vi "Load LV Class from Disk.vi"(8 "error in":errorcluster, 11 "Class Path":path) -> (0 "error out":errorcluster, 3 "Object Out":refnum<class>)   [LabVIEW 2015, in "Configuration Tool.lvlib"]
uses:
  Configuration Tool.lvlib
  <vilib>/NI/Configuration Framework/class discovery singleton/class discovery singleton.lvlib
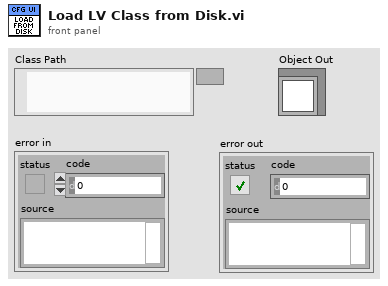
[diagram p1: front panel]
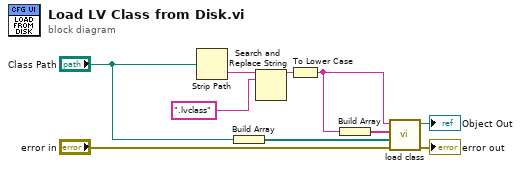
[diagram p0: block diagram]
diagram:
  n1 = Strip Path(path="Class Path") -> (name=w3:string)  [unwired: 1 out]
  n2 = Build Array("Class Path") -> (w5:path[])
  n3 = Search and Replace String(input string=w3, search string=".lvclass") -> (result string=w8:string)  [unwired: 6 in, 3 out]
  n4 = To Lower Case(string=w8) -> (all lower case string=w1:string)
  n5 = Build Array(w1) -> (w2:string[])
  n6 = call <vilib>:"load class.vi"("error in"="error in", "available class paths"=w5, "available class names"=w2, "Class Name"=w1) -> ("error out"=→"error out":errorcluster, "Object Out"=→"Object Out":refnum<class>)  [unwired: 6 in]
